vi "Read Configuration File.vi"(8 "error in (no error)":errorcluster, 11 "Report Generator In":refnum<class "Report Generator.lvclass">) -> (0 "error out":errorcluster, 3 "Report Generator Out":refnum<class "Report Generator.lvclass">)   [LabVIEW 2020, in "Report Generator.lvclass"]
doc: "Load configuration from file. This VI needs to be called before the process is started to have any effect."
uses:
  Report Generator.lvclass
  C:/Users/anton/Documents/GitHub/LUnit/source/Application Framework/Process Classes/Process/Process.lvclass
  Application Framework/Process Classes/Process/Process.lvclass/Process.ctl
  Application Framework/Process Classes/Process/Process.lvclass
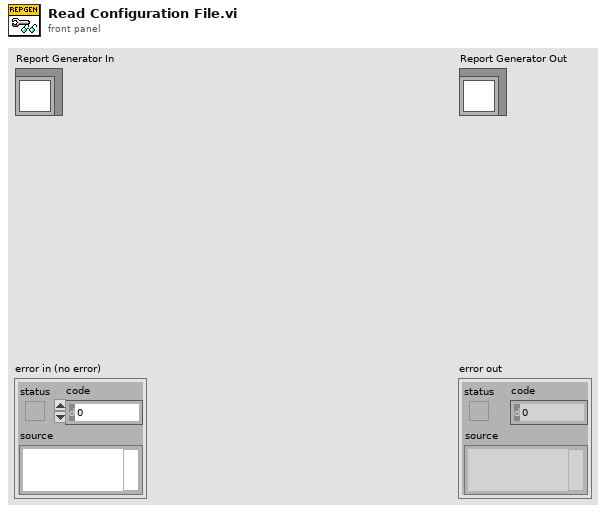
[diagram p1: front panel]
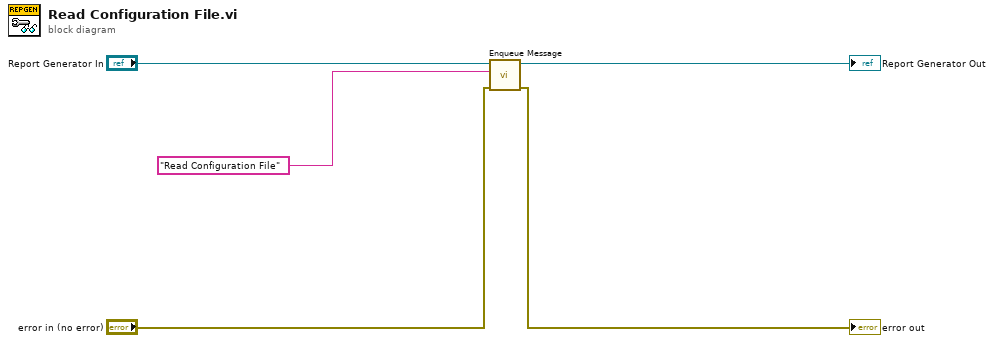
[diagram p0: block diagram]
diagram:
  n1 = call "Enqueue Message.vi"("error in (no error)"="error in (no error)", "Message"="Read Configuration File", "Process In"="Report Generator In") -> ("error out"=→"error out":errorcluster, "Process Out"=→"Report Generator Out":refnum<class "Report Generator.lvclass">)  [unwired: 7 in]
